vi "Create from Config.vi"(8 "error in (no error)":errorcluster, 10 "Config":refnum<class "Task.lvclass">, 11 "Task in":refnum<class "Task.lvclass">) -> (0 "error out":errorcluster, 3 "Task out":refnum<class "Task.lvclass">)   [LabVIEW 2020, in "Volatus.lvlib" / "Task.lvclass"]
uses:
  Task.lvclass
  Task.lvclass/Task.ctl
  VolatusConfig/Task/Task.lvclass
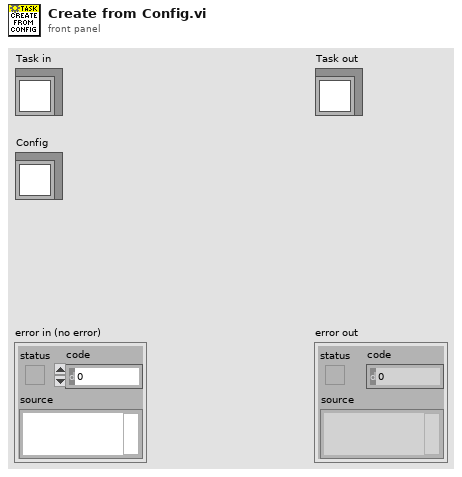
[diagram p1: front panel]
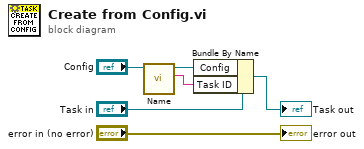
[diagram p0: block diagram]
diagram:
  n1 = call "Name.vi"("Task in"="Config") -> ("Name"=w1:string, "Task out"=w2:refnum<class "Task.lvclass">)  [unwired: 8 in, 1 out]
  n2 = Bundle By Name(cluster="Task in", "Config"=w2, "Task ID"=w1) -> (→"Task out":refnum<class "Task.lvclass">)
  "error out" <- "error in (no error)"
